vi "Integrator Start-Stop.vi"(8 "error in (no error)":errorcluster, 9 "Start/Stop (F: Stop)":bool, 10 "Element (All: 0)":T1(ring), 11 "Yokogawa WT500 in":refnum<class "Yokogawa WT500.lvclass">) -> (0 "error out":errorcluster, 2 "VISA session":refnum<visa-resource-name>, 3 "Yokogawa WT500 out":refnum<class "Yokogawa WT500.lvclass">)   [LabVIEW 2013, in "Universal Power Meter.lvlib" / "Yokogawa WT500.lvlib" / "Yokogawa WT500.lvclass"]
uses:
  Yokogawa WT500.lvclass
  Universal Power Meter class/Universal Power Meter.lvclass
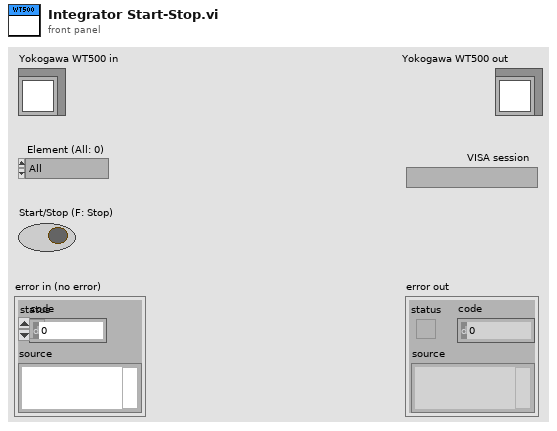
[diagram p1: front panel]
types:
  T1 = enum16{"All", "Element 1", "Element 2", "Element 3", "Element 4", "Element 5", "Element 6"}
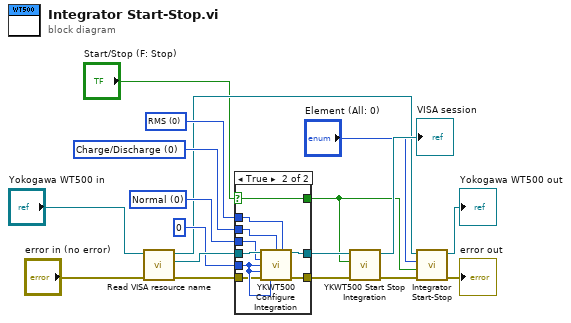
[diagram p0: block diagram]
diagram:
  w13 = u16 0 items=["Charge/Discharge", "Sold/Bought"] ("WP Type (0: Charge/Discharge)")
  w14 = u16 0 items=["RMS", "MEAN", "DC", "R-MEAN", "AC"] ("Q Mode (2: DC)")
  w16 = u16 0 items=["Normal", "Continuous", "R-Normal", "R-Continuous"] ("Integration Mode (0: Normal)")
  n1 = call-dynamic "Read VISA resource name.vi"("error in (no error)"="error in (no error)", "Generic Instrument in"="Yokogawa WT500 in") -> ("error out"=w8:errorcluster, "VISA resource name"=w17:refnum<visa-resource-name>, "Generic Instrument out"=w7:refnum<class "Yokogawa WT500.lvclass">)  [unwired: 7 in]
  n2 = case shown="True" "Start/Stop (F: Stop)" {
    selector: "Start/Stop (F: Stop)" -> [w19 w22]
    tunnel: w17 -> [w21 w30]
    tunnel: w16 -> [_ w29]
    tunnel: 0 ("Integration Time Hour (0)") -> [_ w28]
    tunnel: w14 -> [_ w27]
    tunnel: w13 -> [_ w26]
    tunnel: [w21 w25] -> w11
    tunnel: [w20 w24] -> w10
    tunnel: w8 -> [w20 w23]
    tunnel: [w19 w22] -> w1
    frame False {
    }
    frame True {
      n3 = call <instrlib>:"YKWT500 Configure Integration.vi"("VISA resource name"=w30, "WP Type (0: Charge/Discharge)"=w26, "Q Mode (2: DC)"=w27, "Integration Mode (0: Normal)"=w29, "Integration Time Hour (0)"=w28, "Integration Time Minute (0)"=w28, "error in (no error)"=w23, "Integration Time Second (0)"=w28) -> ("VISA resource name out"=w25:refnum<visa-resource-name>, "error out"=w24:errorcluster)  [unwired: 6 in]
    }
  }
  n4 = call <instrlib>:"YKWT500 Start Stop Integration.vi"("error in (no error)"=w10, "Start/Stop (False: Stop)"=w1, "VISA resource name"=w11) -> ("error out"=w5:errorcluster, "VISA resource name out"=→"VISA session":refnum<visa-resource-name>)  [unwired: 7 in]
  n5 = call-parent "Integrator Start-Stop.vi"("error in (no error)"=w5, "Start/Stop (F: Stop)"=w1, "Element (All: 0)"="Element (All: 0)", "Universal Power Meter in"=w7) -> ("error out"=→"error out":errorcluster, "Universal Power Meter out"=→"Yokogawa WT500 out":refnum<class "Yokogawa WT500.lvclass">)  [unwired: 5 in, 1 out]
